vi "Wait For Current Play To Finish.vi"(8 "error in (no error)":errorcluster, 9 "timeout in ms (-1)":i32=-1, 11 "Visualizer ID":T1) -> (0 "error out":errorcluster, 1 "timed out?":bool)   [LabVIEW 2010, in "Visualizer.lvlib"]
doc: "Given a valid visualizer ID, wait until that visualizer finishes playing the current waveform and then returns. If the visualizer is not currently playing anything, the wait returns immediately."
uses:
  Visualizer.lvlib
  Visualizer Type ID.ctl
  Message.ctl
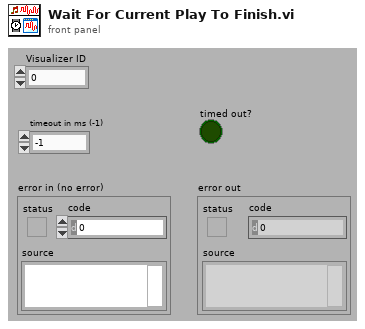
[diagram p1: front panel]
types:
  T1 = typedef "Visualizer.lvlib/Visualizer Type ID.ctl" = u32
  T2 = typedef "Visualizer.lvlib/Message.ctl" = cluster{"Command":string, "Data":variant}
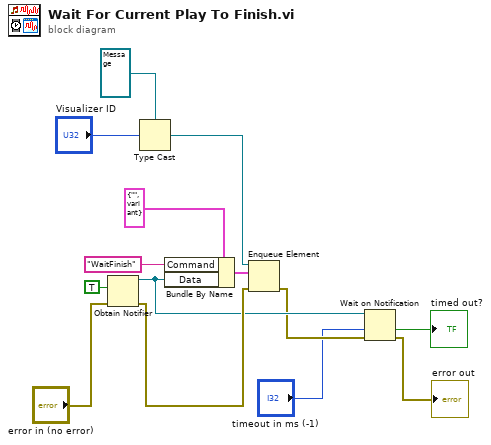
[diagram p0: block diagram]
diagram:
  n1 = Obtain Notifier(notification data type=TRUE, error in (no error)="error in (no error)") -> (notifier out=w5:refnum<notifier>, error out=w6:errorcluster)  [unwired: 2 in, 1 out]
  n2 = Type Cast(type=refnum<queue> refnum ("queue out"), x="Visualizer ID") -> (*(type *) &x=w11:refnum<queue>)
  n3 = Bundle By Name(cluster=T2 {"Command"="", "Data"=variant} ("Message"), "Command"="WaitFinish", "Data"=w5) -> (w14:T2)
  n4 = Enqueue Element(queue=w11, element=w14, error in (no error)=w6) -> (error out=w4:errorcluster)  [unwired: 1 in, 2 out]
  n5 = Wait on Notification(notifier=w5, timeout in ms (-1)="timeout in ms (-1)", error in (no error)=w4) -> (timed out?=→"timed out?":bool, error out=→"error out":errorcluster)  [unwired: 1 in, 2 out]
